vi "Do.vi"(8 "error in (no error)":errorcluster, 10 "DMM":refnum<class "DMM.lvclass">, 11 "Init DMM in":refnum<class "Init DMM.lvclass">) -> (0 "error out":errorcluster, 2 "DMM":refnum<class "DMM.lvclass">, 3 "Init DMM out":refnum<class "Init DMM.lvclass">)   [LabVIEW 2020, in "Init DMM.lvclass"]
uses:
  Init DMM.lvclass
  DMM/DMM.lvclass
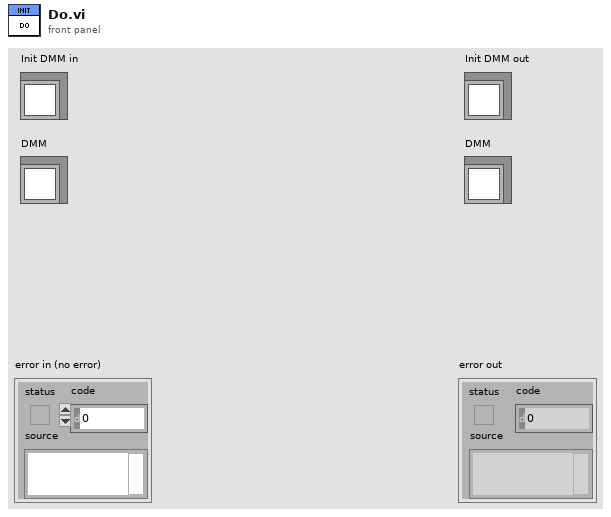
[diagram p1: front panel]
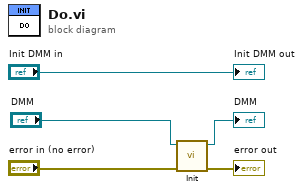
[diagram p0: block diagram]
diagram:
  n1 = call-dynamic "Init.vi"("error in (no error)"="error in (no error)", "DMM in"="DMM") -> ("error out"=→"error out":errorcluster, "DMM out"=→"DMM":refnum<class "DMM.lvclass">)  [unwired: 8 in]
  "Init DMM out" <- "Init DMM in"
